vi "Test.vi"(10 "XSD File Path":path=path "D:/NI/Sales/Canada/Sales/2014/Mon Espace/Modbus Custom-Device/XML Deserializer/Modbus_Custom_Device.xsd", 11 "XML File Path":path=path "D:/NI/Sales/Canada/Sales/2014/Mon Espace/Modbus Custom-Device/XML Deserializer/XML Test Files/Reference_XML_000.xml") -> (0 "error out":errorcluster, 2 "List of Modbus Items":T2[](array[typedef]), 3 "General Settings":T1={"Communication_Type"=0, "Modbus_Type"=0, "Read_Write_Loop_Period"=-1, "TCP Settings"={"TCP_Settings_Port"=0, "TCP_Settings_IP_Timeout"=0, "TCP_Settings_IP_Slave_Address"=""}, "Serial Settings"={"Serial_Settings_Flow_Control"=0, "Serial_Settings_Baud_Rate"=0, "Serial_Settings_Parity"=0, "Serial_Settings_Resource_Name"="", "Serial_Settings_Serial_Type"=0, "Serial_Settings_Unit_ID"=0}} {"Communication_Type" items=["TCP", "Serial"]; "Modbus_Type" items=["Master", "Slave"]; "Serial Settings"."Serial_Settings_Flow_Control" items=["None", "XONXOFF", "RTSCTS", "XONXOFFANDRTSCTS", "DTRDSR", "XONXOFFANDDTRDSR"]; "Serial Settings"."Serial_Settings_Parity" items=["None", "Odd", "Even"]; "Serial Settings"."Serial_Settings_Serial_Type" items=["RTU", "ASCII"]})   [LabVIEW 2014, in "XML_Deserializer.lvlib"]
uses:
  API/XML_Deserializer.lvlib
  API/Controls/Modbus_Items.ctl
  API/Controls/Modbus_Item_Type.ctl
  Shared/Modbus Shared.lvlib
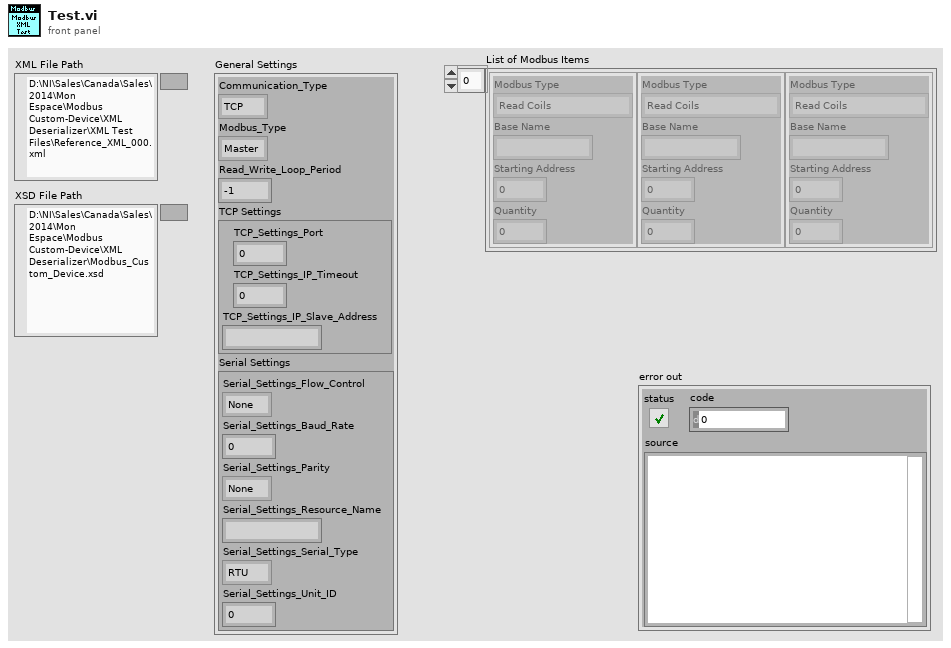
[diagram p1: front panel]
types:
  T1 = cluster{"Communication_Type":i32, "Modbus_Type":i32, "Read_Write_Loop_Period":i64, "TCP Settings":cluster{"TCP_Settings_Port":u16, "TCP_Settings_IP_Timeout":u32, "TCP_Settings_IP_Slave_Address":string}, "Serial Settings":cluster{"Serial_Settings_Flow_Control":i32, "Serial_Settings_Baud_Rate":u32, "Serial_Settings_Parity":i32, "Serial_Settings_Resource_Name":string, "Serial_Settings_Serial_Type":i32, "Serial_Settings_Unit_ID":i8}}
  T2 = typedef "Modbus Shared.lvlib/Modbus_Items.ctl" = cluster{"Modbus Type":T3, "Base Name":string, "Starting Address":u16, "Quantity":u16}
  T3 = typedef "Modbus Shared.lvlib/Modbus_Item_Type.ctl" = enum16{"Read Coils", "Read Discrete Inputs", "Read Holding Registers", "Read Input Registers", "Write Multiple Coils", "Write Multiple Holding Registers", "Write Single Coil", "Write Single Holding Register", "Write Multiple Discrete Inputs", "Write Multiple Input Registers"}
  T4 = typedef "Modbus Shared.lvlib/Modbus_General_Settings.ctl" = cluster{"Communication_Type":T5, "Modbus_Type":T6, "Read_Write_Loop_Period":i64, "TCP Settings":cluster{"TCP_Settings_Port":u16, "TCP_Settings_IP_Timeout":u32, "TCP_Settings_IP_Slave_Address":string}, "Serial Settings":cluster{"Serial_Settings_Flow_Control":T7, "Serial_Settings_Baud_Rate":u32, "Serial_Settings_Parity":T8, "Serial_Settings_Resource_Name":string, "Serial_Settings_Serial_Type":T9, "Serial_Settings_Unit_ID":u8}}
  T5 = typedef "Modbus Shared.lvlib/Modbus_Communication_Type.ctl" = i32
  T6 = typedef "Modbus Shared.lvlib/Modbus_Type.ctl" = i32
  T7 = typedef "Modbus Shared.lvlib/Modbus_Serial_Settings_Flow_Control.ctl" = i32
  T8 = typedef "Modbus Shared.lvlib/Modbus_Serial_Settings_Parity.ctl" = i32
  T9 = typedef "Modbus Shared.lvlib/Modbus_Serial_Settings_Serial_Type.ctl" = i32
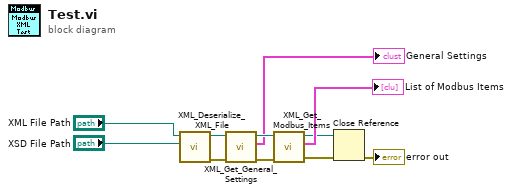
[diagram p0: block diagram]
diagram:
  n1 = call "XML_Deserialize_XML_File.vi"("XSD Path"="XSD File Path", "XML Path"="XML File Path") -> ("error out"=w1:errorcluster, "reference out"=w2:refnum<k24>)  [unwired: 8 in]
  n2 = call "XML_Get_General_Settings.vi"("error in (no error)"=w1, ".NET Refnum in"=w2) -> ("error out"=w6:errorcluster, "General Settings"=→"General Settings":T4, ".NET Refnum out"=w5:refnum<k24>)  [unwired: 7 in]
  n3 = call "XML_Get_Modbus_Items.vi"("error in (no error)"=w6, "reference out"=w5) -> ("error out"=w7:errorcluster, "Array"=→"List of Modbus Items":T2[], "reference out"=w8:refnum<k24>)  [unwired: 7 in]
  n4 = Close Reference(reference=w8, error in (no error)=w7) -> (error out=→"error out":errorcluster)
